vi "Create_VI_Fpterm_Images.vi"(7 "All Controls?":bool, 8 "error in (no error)":errorcluster, 9 "Image Depth":i32=24, 10 "Image Format (jpeg)":enum32{"PNG", "JPEG", "GIF"}(ring)=enum."JPEG", 11 "VI":refnum<vi>) -> (0 "error out":errorcluster, 2 "HTML File Path":path, 3 "Directory for images":path)   [LabVIEW 2020, in "NI_ReportGenerationCore.lvlib"]
uses:
  <vilib>/Utility/NIReport.llb/NI_ReportGenerationCore.lvlib
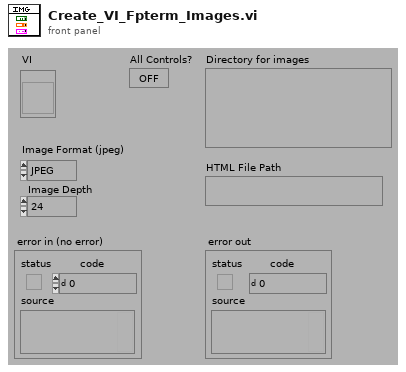
[diagram p1: front panel]
types:
  T1 = cluster{"Printing:Custom All Controls?":bool, "Printing:Custom Connector?":bool, "Printing:Custom Control Descriptions?":bool, "Printing:Custom Control Types?":bool, "Printing:Custom Controls?":bool, "Printing:Custom Description?":bool, "Printing:Custom Diagram Hidden?":bool, "Printing:Custom Diagram Repeat?":bool, "Printing:Custom Diagram?":bool, "Printing:Custom Hierarchy?":bool, "Printing:Custom History?":bool, "Printing:Custom Panel Border?":bool, "Printing:Custom Panel?":bool, "Printing:Custom SubVIs?":bool}
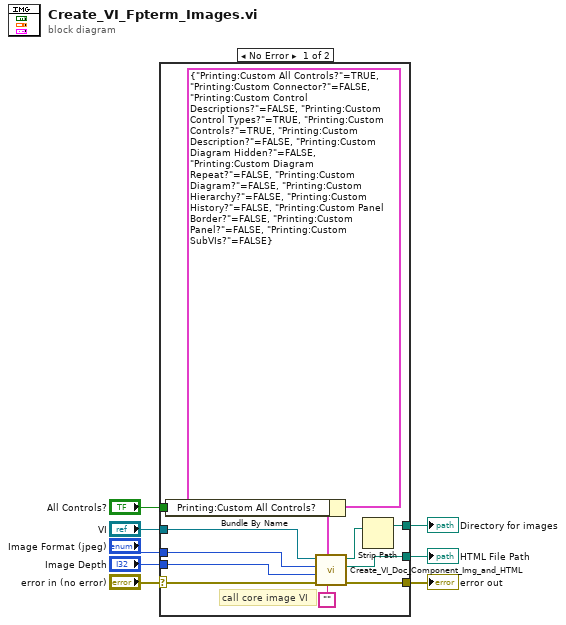
[diagram p0: block diagram]
diagram:
  n1 = case shown="No Error" "error in (no error)" {
    selector: "error in (no error)" -> [w10 w21]
    tunnel: "VI" -> [w20 _]
    tunnel: "Image Format (jpeg)" -> [w19 _]
    tunnel: "Image Depth" -> [w18 _]
    tunnel: [w17 w21] -> w5
    tunnel: [w14 _] -> w4
    tunnel: [w13 _] -> w3
    tunnel: "All Controls?" -> [w11 _]
    frame No Error {
      # "call core image VI"
      n2 = Bundle By Name(cluster=T1 {"Printing:Custom All Controls?"=TRUE, "Printing:Custom Connector?"=FALSE, "Printing:Custom Control Descriptions?"=FALSE, "Printing:Custom Control Types?"=TRUE, "Printing:Custom Controls?"=TRUE, "Printing:Custom Description?"=FALSE, "Printing:Custom Diagram Hidden?"=FALSE, "Printing:Custom Diagram Repeat?"=FALSE, "Printing:Custom Diagram?"=FALSE, "Printing:Custom Hierarchy?"=FALSE, "Printing:Custom History?"=FALSE, "Printing:Custom Panel Border?"=FALSE, "Printing:Custom Panel?"=FALSE, "Printing:Custom SubVIs?"=FALSE} ("Content Options"), "Printing:Custom All Controls?"=w11) -> (w12:T1)
      n3 = call <vilib>:"Create_VI_Doc_Component_Img_and_HTML.vi"("special chars in file path of image"="", "Content Options"=w12, "error in (no error)"=w10, "Image Depth"=w18, "Image Format (jpeg)"=w19, "VI"=w20) -> ("error out"=w17:errorcluster, "HTML File Path"=w13:path, "Path to image"=w15:path)  [unwired: 3 in]
      n4 = Strip Path(path=w15) -> (stripped path=w14:path)  [unwired: 1 out]
    }
    frame Error {
    }
  }
  "error out" <- w5
  "Directory for images" <- w4
  "HTML File Path" <- w3
